vi "Configure Motion Magic.vi"(8 "error in (no error)":errorcluster, 11 "Motion Magic Parameters":T1) -> (0 "error out":errorcluster)   [LabVIEW 2017, in "Drive Train.lvlib"]
uses:
  Drive Train.lvlib
  Controls/FGV Actions.ctl
  <vilib>/Rock Robotics/WPI/ThirdParty/Phoenix-LabVIEW/Motor Controller/Controls/CTRE_Phoenix_MotorControl_ControlMode.ctl
  Controls/Motion Magic Parameters.ctl
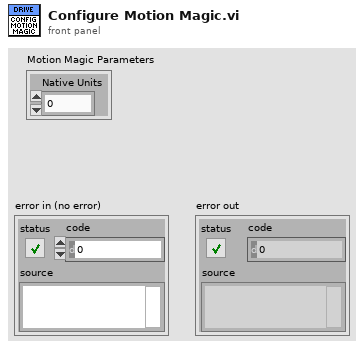
[diagram p1: front panel]
types:
  T1 = typedef "Drive Train.lvlib/Motion Magic Parameters.ctl" = cluster{"Native Units":dbl}
  T2 = typedef "Drive Train.lvlib/FGV Actions.ctl" = enum16{"Get", "Set"}
  T3 = typedef "CTRE_Phoenix_MotorControl_ControlMode.ctl" = u16
  T4 = typedef "Drive Train.lvlib/Library Information.ctl" = cluster{"Right Motor Name":string, "Left Motor Name":string, "Current Control Mode":T3, "Motion Magic Parameters":T1, "Motor Controllers Parameters":T5}
  T5 = typedef "Drive Train.lvlib/Motor Controllers Parameters.ctl" = cluster{"Max Current (amps)":i32, "PID Buckets":cluster{"High Gear":i32, "High Gear Ramp":i32, "Low Gear":i32, "Low Gear Ramp":i32}}
  T6 = typedef "WPI_MotorControlDeviceRef.ctl" = cluster{"DeviceStatus":errorcluster, "Type":T7, "PWM":cluster{"PWM Channel":T8, "DeadBand":T9}, "CAN":cluster{"Device Number":u8, "SetOutput VI Ref":variant, "GetOutput VI Ref":variant, "Enable VI Ref":variant, "Disable VI Ref":variant, "Data":variant}, "Invert":bool, "DIO PWM":cluster{"PWM \"Enable\" Channel":T8, "DIOChannel":T10, "PWM Rate":dbl}}
  T7 = typedef "WPI_MotorControlType.ctl" = enum16{"PWM", "CAN", "DIO PWM"}
  T8 = typedef "FPGA_DIOPWMChannel.ctl" = enum8{"PWM 0", "PWM 1", "PWM 2", "PWM 3", "PWM 4", "PWM 5", "PWM 6", "PWM 7", "PWM 8", "PWM 9", "PWM MXP 0", "PWM MXP 1", "PWM MXP 2", "PWM MXP 3", "PWM MXP 4", "PWM MXP 5", "PWM MXP 6", "PWM MXP 7", "PWM MXP 8", "PWM MXP 9", "Invalid"}
  T9 = typedef "WPI_PWMDeadband.ctl" = cluster{"Name":string, "maxPositivePwm":i32, "minPositivePwm":i32, "centerPwm":i32, "maxNegativePwm":i32, "minNegativePwm":i32, "angularRange":u16}
  T10 = typedef "FPGA_DIOChannel.ctl" = enum8{"DIO 0", "DIO 1", "DIO 2", "DIO 3", "DIO 4", "DIO 5", "DIO 6", "DIO 7", "DIO 8", "DIO 9", "DIO MXP 0", "DIO MXP 1", "DIO MXP 2", "DIO MXP 3", "DIO MXP 4", "DIO MXP 5", "DIO MXP 6", "DIO MXP 7", "DIO MXP 8", "DIO MXP 9", "DIO MXP 10", "DIO MXP 11", "DIO MXP 12", "DIO MXP 13", "DIO MXP 14", "DIO MXP 15", "SPI Port CS1", "SPI Port CS2", "SPI Port CS3", "SPI Port MISO", "SPI Port MOSI", "Invalid"}
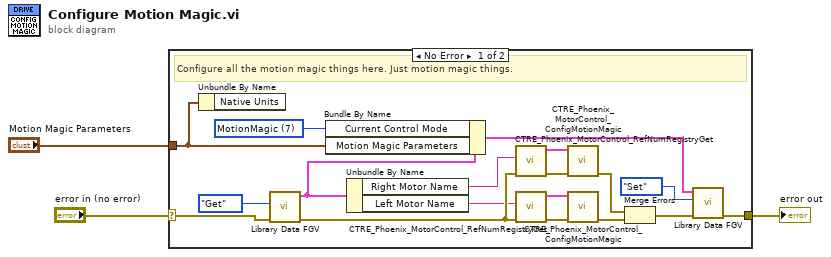
[diagram p0: block diagram]
diagram:
  n1 = case shown="No Error" "error in (no error)" {
    selector: "error in (no error)" -> [w21 w22]
    tunnel: [w14 w22] -> w2
    tunnel: "Motion Magic Parameters" -> [w4 _]
    frame No Error {
      w11 = T3 7 items=["PercentOutput"=0, "Position"=1, "Velocity"=2, "Current"=3, "Follower"=5, "MotionProfile"=6, "MotionMagic"=7, "MotionMagicArc"=8, "MotionProfileArc"=10, "Disabled"=15] ("Control Mode")
      # "Configure all the motion magic things here. Just motion magic things."
      n2 = Unbundle By Name(w4) -> ()  [unwired: 1 out]
      n3 = call "Library Data FGV.vi"("error in (no error)"=w21, "FGV Actions"=FGV_Actions."Get") -> ("error out"=w19:errorcluster, "Library Information out"=w13:T4)  [unwired: 8 in]
      n4 = Bundle By Name(cluster=w13, "Current Control Mode"=w11, "Motion Magic Parameters"=w4) -> (w12:T4)
      n5 = Unbundle By Name(w13) -> ("Right Motor Name"=w17:string, "Left Motor Name"=w18:string)
      n6 = call <vilib>:"CTRE_Phoenix_MotorControl_RefNumRegistryGet.vi"("error in (no error)"=w19, "refnum name"=w17) -> ("error out"=w9:errorcluster, "PhoenixMotorControlDevRef"=w6:T6)  [unwired: 8 in]
      n7 = call <vilib>:"CTRE_Phoenix_MotorControl_RefNumRegistryGet.vi"("error in (no error)"=w19, "refnum name"=w18) -> ("error out"=w10:errorcluster, "PhoenixMotorControlDevRef"=w5:T6)  [unwired: 8 in]
      n8 = call <vilib>:"CTRE_Phoenix_MotorControl_ConfigMotionMagic.vi"("error in (no error)"=w9, "PhoenixMotorControlDevRef"=w6) -> ("error out"=w8:errorcluster)  [unwired: 8 in, 1 out]
      n9 = call <vilib>:"CTRE_Phoenix_MotorControl_ConfigMotionMagic.vi"("error in (no error)"=w10, "PhoenixMotorControlDevRef"=w5) -> ("error out"=w7:errorcluster)  [unwired: 8 in, 1 out]
      n10 = Merge Errors(w8, w7) -> (w15:errorcluster)
      n11 = call "Library Data FGV.vi"("error in (no error)"=w15, "FGV Actions"=FGV_Actions."Set", "Library Information in"=w12) -> ("error out"=w14:errorcluster)  [unwired: 7 in, 1 out]
    }
    frame Error {
    }
  }
  "error out" <- w2
